vi "WFS Get Line.vi"(8 "error in (no error)":errorcluster {"code" format="%.0x"}, 10 "Line":i32 format="%.0g", 11 "instrument handle":refnum<visa-resource-name>) -> (0 "error out":errorcluster {"code" format="%.0x"}, 2 "Line Selected":sgl[](array[numeric]) format="%.2p", 3 "instrument handle out":refnum<visa-resource-name>)   [LabVIEW 2020]
doc: "This VI returns a single horizontal line of the image in a linear array.\n\nNote: This VI is not available in Highspeed Mode!"
uses:
  WFS_32.dll
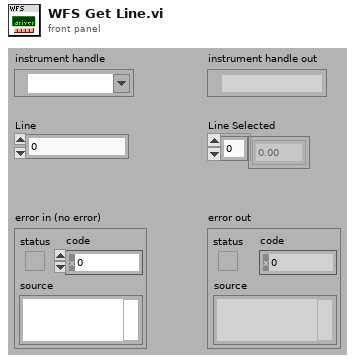
[diagram p1: front panel]
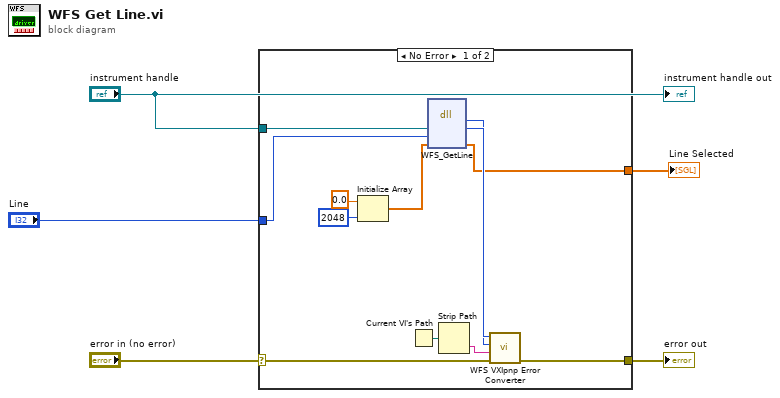
[diagram p0: block diagram]
diagram:
  n1 = case shown="No Error" "error in (no error)" {
    selector: "error in (no error)" -> [w12 w18]
    tunnel: [w11 w18] -> w5
    tunnel: "instrument handle" -> [w16 _]
    tunnel: "Line" -> [w10 _]
    tunnel: [w6 _] -> w1
    frame No Error {
      n2 = Initialize Array(sgl 0.0 ("element"), 2048 ("dimension size")) -> (w9:sgl[])
      n3 = Current VI's Path() -> (path=w17:path)
      n4 = dll-call lib="WFS_*.*" fn="WFS_GetLine"("Instrument Handle"=w16, "Line"=w10, "Line Selected"=w9) -> (w14:i32, "Instrument Handle"=w15:u32, "Line Selected"=w6:sgl[])  [unwired: 4 in, 2 out]
      n5 = Strip Path(path=w17) -> (name=w13:string)  [unwired: 1 out]
      n6 = call "WFS VXIpnp Error Converter.vi"("error in (no error)"=w12, "Name Of VI (\"\")"=w13, "CVI Error Code (0)"=w14, "instrument handle"=w15) -> ("error out"=w11:errorcluster)  [unwired: 6 in, 1 out]
    }
    frame Error {
    }
  }
  "error out" <- w5
  "Line Selected" <- w1
  "instrument handle out" <- "instrument handle"
